vi "Report_Create.vi"(8 "error in (no error)":errorcluster, 9 "appended array 2":refnum<vi>[](array[refnum]), 10 "output cluster":T1, 11 "Save Filename":path=path "C:/tmp") -> (0 "error out":errorcluster)   [LabVIEW 2010]
uses:
  <vilib>/Utility/NIReport.llb/NI_report.lvclass
  <vilib>/Utility/NIReport.llb/Append Text Table to Report (wrap).vi
  <vilib>/Utility/NIReport.llb/Append Report Text (str wrap).vi
panel:
  out "File path":path
  in  "printer name (default) or file path (dialog)":string="PDFCreator"
  in  "report type":T2(ring)
  in  "font settings":T3={"charset (-1)"=-1, "weight (-1)"=-1, "name"="", "size"="12"}
  in  "orientation (portrait)":u16(ring) items=["portrait", "landscape"]
  in  "footers":T4
  in  "margins":T5={"margins (1.00)"={"top"=1.0, "left"=1.0, "right"=1.0, "bottom"=1.0}, "measurement system (default)"=0} {"measurement system (default)" items=["Default", "US", "Metric"]; "margins (1.00)"."right" format="%0.2f"; "margins (1.00)"."bottom" format="%0.2f"; "margins (1.00)"."top" format="%0.2f"; "margins (1.00)"."left" format="%0.2f"}
  in  "headers":T4
  in  "text to be printed":string="Проверка генератора отчетов"
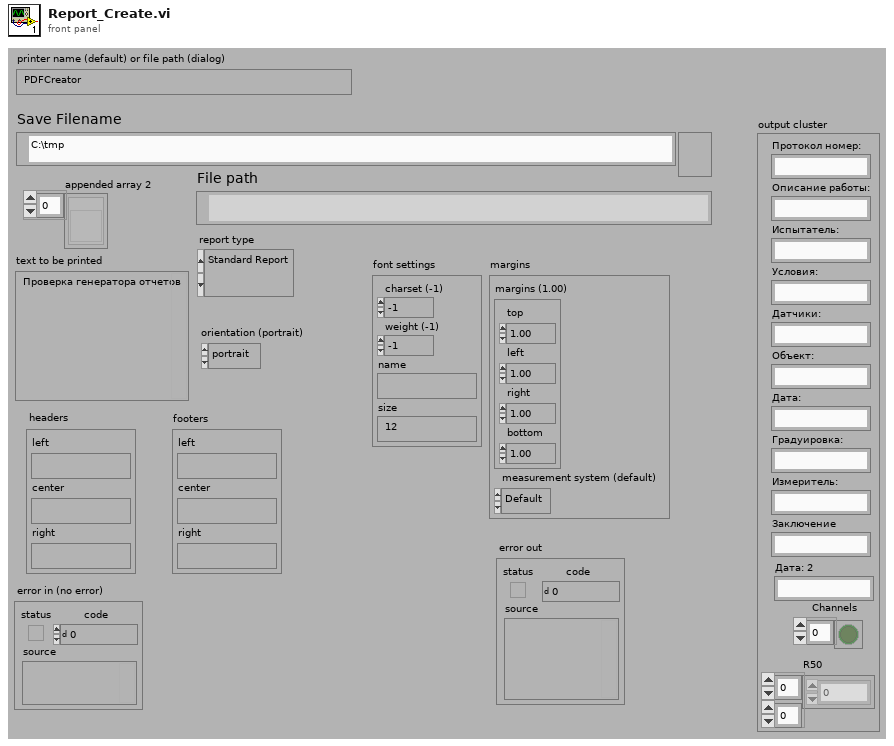
[diagram p1: front panel]
types:
  T1 = cluster{"Протокол номер:":string, "Описание работы:":string, "Испытатель:":string, "Условия:":string, "Датчики:":string, "Объект:":string, "Дата:":string, "Градуировка:":string, "Измеритель:":string, "Заключение":string, "Дата: 2":string, "Channels":bool[], "R50":dbl[][]}
  T2 = enum16{"Standard Report", "HTML", "Word", "Excel"}
  T3 = cluster{"charset (-1)":i16, "weight (-1)":i16, "name":string, "size":string}
  T4 = cluster{"left":string, "center":string, "right":string}
  T5 = cluster{"margins (1.00)":cluster{"top":dbl, "left":dbl, "right":dbl, "bottom":dbl}, "measurement system (default)":u16}
  T6 = cluster{"top":dbl, "left":dbl, "right":dbl, "bottom":dbl}
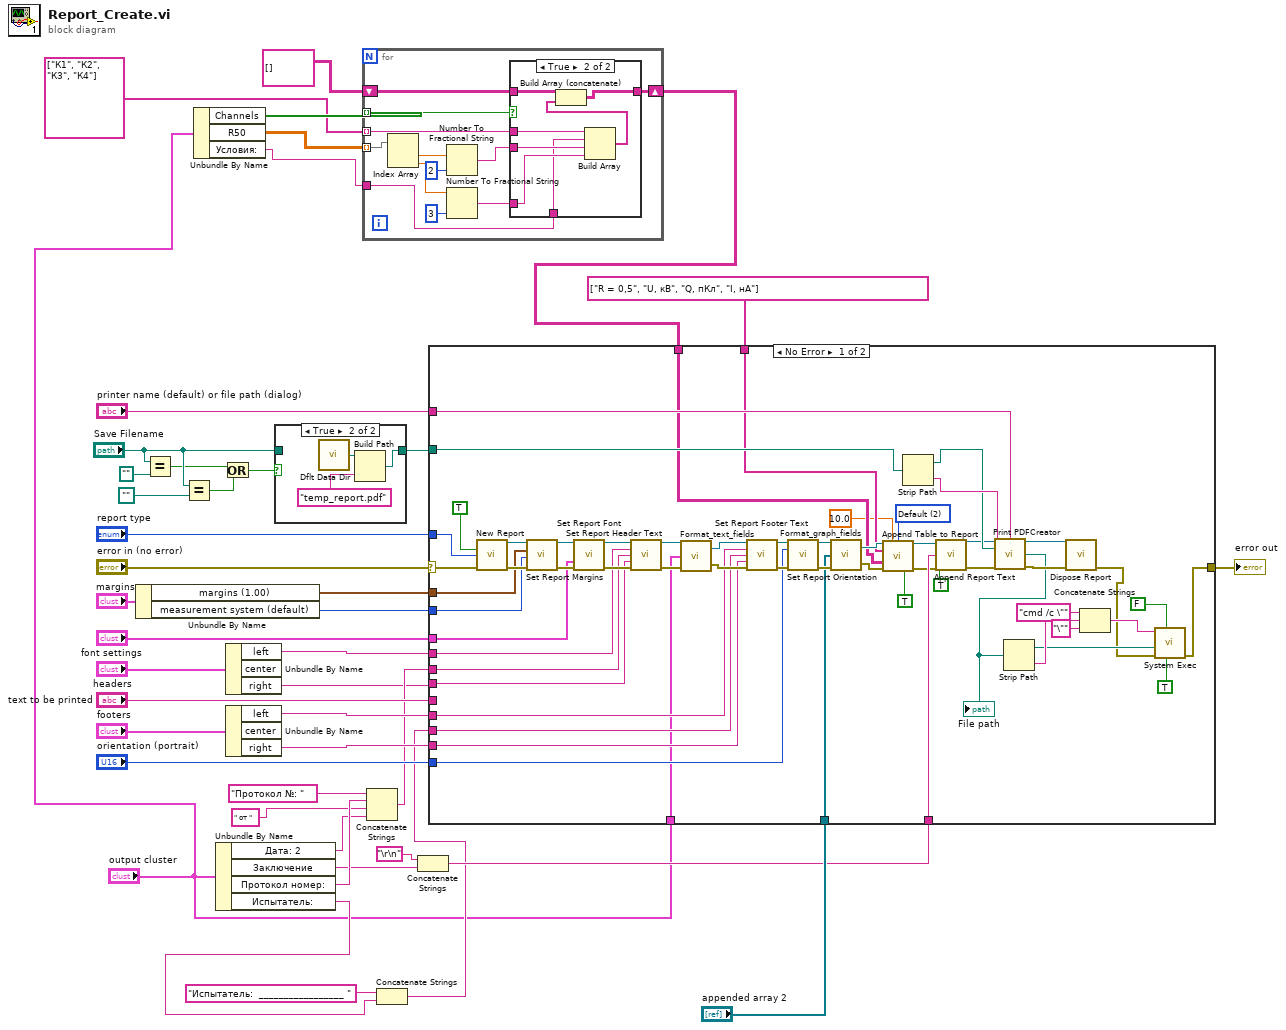
[diagram p0: block diagram]
diagram:
  n1 = Unbundle By Name("margins") -> ("margins (1.00)"=w41:T6, "measurement system (default)"=w40:u16)
  n2 = Equal?(x="Save Filename", y=path "") -> (x = y?=w12:bool)
  n3 = Equal?(x="Save Filename", y=path "") -> (x = y?=w13:bool)
  n4 = Unbundle By Name("output cluster") -> ("Channels"=w6:bool[], "R50"=w2:dbl[][], "Условия:"=w1:string)
  n5 = Unbundle By Name("output cluster") -> ("Дата: 2"=w9:string, "Заключение"=w23:string, "Протокол номер:"=w26:string, "Испытатель:"=w19:string)
  n6 = Or(x=w12, y=w13) -> (x .or. y?=w11:bool)
  n7 = Unbundle By Name("headers") -> ("left"=w38:string, "right"=w10:string)  [unwired: 1 out]
  n8 = Unbundle By Name("footers") -> ("left"=w36:string, "right"=w35:string)  [unwired: 1 out]
  n9 = case shown="True" w11 {
    tunnel: "Save Filename" -> [w44 _]
    tunnel: [w44 w45] -> w16
    frame False {
    }
    frame True {
      n10 = call <vilib>:"Dflt Data Dir.vi"() -> ("App:Default Data Directory"=w47:path)
      n11 = Build Path(base path=w47, name or relative path="temp_report.pdf") -> (appended path=w45:path)
    }
  }
  n12 = for {
    tunnel: w6 -> [w59] mode=indexing
    shift-right: [w56] -> w4
    shift-left: string[][] [] -> [w57]
    tunnel: string[] ["К1", "К2", "К3", "К4"] -> [w58] mode=indexing
    tunnel: w2 -> [w55] mode=indexing
    tunnel: w1 -> [w50]
    n13 = Index Array(array=w55) -> (element #1=w52:dbl, element #2=w54:dbl)  [unwired: 2 in]
    n14 = Number To Fractional String(number=w52, precision (6)=i16 2) -> (F-format string=w51:string)  [unwired: 2 in]
    n15 = Number To Fractional String(number=w54, precision (6)=i16 3) -> (F-format string=w53:string)  [unwired: 2 in]
    n16 = case shown="True" w59 {
      tunnel: w58 -> [_ w62]
      tunnel: w57 -> [w60 w67]
      tunnel: [w60 w66] -> w56
      tunnel: w53 -> [_ w64]
      tunnel: w51 -> [_ w63]
      tunnel: w50 -> [_ w61]
      frame False {
      }
      frame True {
        n17 = Build Array(w62, w61, w63, w64) -> (w65:string[])
        n18 = Build Array (concatenate)(w67, w65) -> (w66:string[][])
      }
    }
  }
  n19 = Concatenate Strings("Протокол №: ", w26, " от ", w9) -> (w25:string)
  n20 = Concatenate Strings("Испытатель:  _________________ ", w19) -> (w18:string)
  n21 = Concatenate Strings("\r\n", w23) -> (w22:string)
  n22 = case shown="No Error" "error in (no error)" {
    selector: "error in (no error)" -> [w115 w126]
    tunnel: [w88 w126] -> w43
    tunnel: w41 -> [w123 _]
    tunnel: w40 -> [w120 _]
    tunnel: w38 -> [w112 _]
    tunnel: w25 -> [w119 _]
    tunnel: w10 -> [w118 _]
    tunnel: w36 -> [w108 _]
    tunnel: w18 -> [w106 _]
    tunnel: w35 -> [w107 _]
    tunnel: "text to be printed" -> [_ _]
    tunnel: "orientation (portrait)" -> [w102 _]
    tunnel: "font settings" -> [w105 _]
    tunnel: "report type" -> [w101 _]
    tunnel: "printer name (default) or file path (dialog)" -> [w98 _]
    tunnel: w16 -> [w86 _]
    tunnel: "output cluster" -> [w84 _]
    tunnel: w22 -> [w80 _]
    tunnel: "appended array 2" -> [w78 _]
    tunnel: string[] ["R = 0,5", "U, кВ", "Q, пКл", "I, нА"] -> [w72 _]
    tunnel: w4 -> [w71 _]
    frame No Error {
      w70 = u16 2 items=["US", "Metric", "Default"] ("measurement system")
      n23 = call <vilib>:"New Report.vi"("display alerts? (F)"=TRUE, "report type"=w101, "error in (no error)"=w115) -> ("report out"=w125:refnum<class "NI_report.lvclass">, "error out"=w124:errorcluster)  [unwired: 3 in, 8 out]
      n24 = call-dynamic "Set Report Margins.vi"("report in"=w125, "margins (1.00)"=w123, "measurement system (default)"=w120, "error in (no error)"=w124) -> ("report out"=w117:refnum<class "NI_report.lvclass">, "error out"=w116:errorcluster)  [unwired: 10 out]
      n25 = call-dynamic "Set Report Font.vi"("report in"=w117, "font settings"=w105, "error in (no error)"=w116) -> ("report out"=w122:refnum<class "NI_report.lvclass">, "error out"=w121:errorcluster)  [unwired: 3 in, 8 out]
      n26 = call-dynamic "Set Report Header Text.vi"("report in"=w122, "left header text"=w112, "center header text"=w119, "right header text"=w118, "error in (no error)"=w121) -> ("report out"=w114:refnum<class "NI_report.lvclass">, "error out"=w109:errorcluster)  [unwired: 2 in, 7 out]
      n27 = call "Format_text_fields.vi"("error out"=w109, "output cluster"=w84, "report out 2"=w114) -> ("error out 2"=w110:errorcluster, "report out"=w113:refnum<class "NI_report.lvclass">)
      n28 = call-dynamic "Set Report Footer Text.vi"("report in"=w113, "left footer text"=w108, "center footer text"=w106, "right footer text"=w107, "error in (no error)"=w110) -> ("report out"=w104:refnum<class "NI_report.lvclass">, "error out"=w103:errorcluster)  [unwired: 1 in, 8 out]
      n29 = call-dynamic "Set Report Orientation.vi"("report in"=w104, "orientation (portrait)"=w102, "error in (no error)"=w103) -> ("report out"=w97:refnum<class "NI_report.lvclass">, "error out"=w83:errorcluster)  [unwired: 11 out]
      n30 = call "Format_graph_fields.vi"("error out 2"=w83, "appended array 2"=w78, "report out 2"=w97) -> ("error out"=w76:errorcluster, "report out"=w77:refnum<class "NI_report.lvclass">)
      n31 = call-poly <vilib>:"Append Table to Report.vi"("report in"=w77, "column width (1)"=10.0, "measurement system"=w70, "column headers"=w72, "text data"=w71, "error in (no error)"=w76, "show grid lines"=TRUE) -> ("report out"=w74:refnum<class "NI_report.lvclass">, "error out"=w75:errorcluster)  [unwired: 5 in, 2 out]
      n32 = Strip Path(path=w86) -> (stripped path=w85:path, name=w87:string)
      n33 = call-poly <vilib>:"Append Report Text.vi"("report in"=w74, "text"=w80, "append on new line? (F)"=TRUE, "error in (no error)"=w75) -> ("report out"=w81:refnum<class "NI_report.lvclass">, "error out"=w82:errorcluster)  [unwired: 2 in, 8 out]
      n34 = call "Print PDFCreator.vi"("report in"=w81, "Printer name"=w98, "Save Directory"=w85, "Save Filename"=w87, "error in (no error)"=w82) -> ("report out"=w99:refnum<class "NI_report.lvclass">, "File path"=w90:path, "error out"=w100:errorcluster)  [unwired: 8 out]
      "File path" <- w90
      n35 = Strip Path(path=w90) -> (stripped path=w93:path, name=w94:string)
      n36 = call-dynamic "Dispose Report.vi"("report in"=w99, "error in (no error)"=w100) -> ("error out"=w89:errorcluster)  [unwired: 3 in, 10 out]
      n37 = Concatenate Strings("cmd /c \"" ("string"), w94, "\"" ("string")) -> (w95:string)
      n38 = call <vilib>:"System Exec.vi"("run minimized? (F)"=TRUE, "wait until completion? (T)"=FALSE, "error in (no error)"=w89, "working directory"=w93, "command line"=w95) -> ("error out"=w88:errorcluster)  [unwired: 3 in, 3 out]
    }
    frame Error {
    }
  }
  "error out" <- w43
